vi "4wireRes.vi"(5 "Settling time":dbl=2.0, 7 "Enable Output (T: Enable)":bool, 8 "error in (no error)":errorcluster, 10 "VISA nanoVM":refnum<visa-resource-name>="nanovoltmeter", 11 "VISA current":refnum<visa-resource-name>="K2401") -> (0 "R4pt":dbl, 1 "R2pt":sgl, 2 "error out":errorcluster, 3 "VISA nanovoltmeter out":refnum<visa-resource-name>, 6 "VISA current out":refnum<visa-resource-name>)   [LabVIEW 2019]
uses:
  _Global variables 1.vi
  <instrlib>/Keithley 2182/Keithley 2182.lvlib
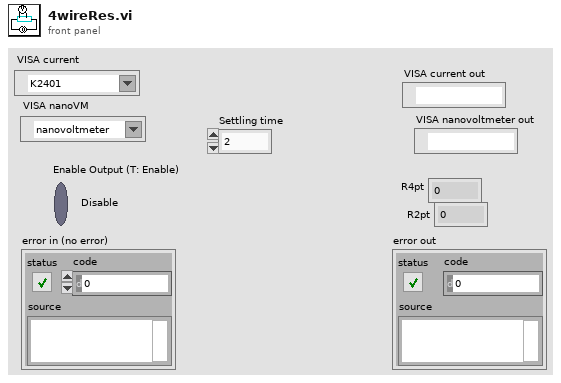
[diagram p1: front panel]
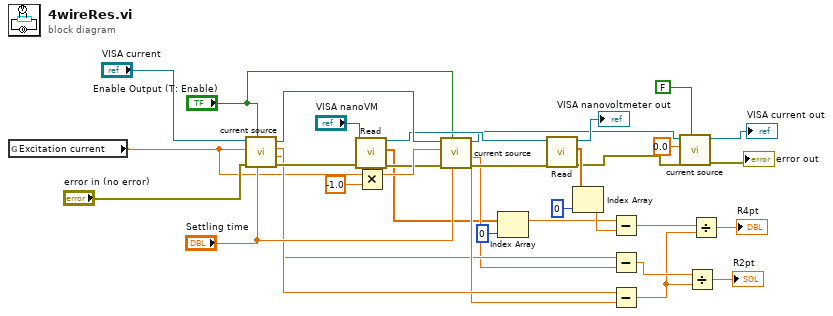
[diagram p0: block diagram]
diagram:
  n1 = global read "_Global variables 1.vi" "Excitation current"() -> (w1:dbl)
  n2 = call "current source.vi"("Settling time"="Settling time", "Enable Output (T: Enable)"="Enable Output (T: Enable)", "error in (no error)"="error in (no error)", "Output Level (0)"=w1, "VISA current"="VISA current") -> ("error out"=w33:errorcluster, "Voltage"=w22:sgl, "Current"=w24:sgl, "VISA resource name out"=w29:refnum<visa-resource-name>)  [unwired: 3 in]
  n3 = call <instrlib>:"Read.vi"("error in (no error)"=w33, "VISA resource name"="VISA nanoVM") -> ("error out"=w28:errorcluster, "Measurements"=w20:dbl[], "VISA resource name out"=w25:refnum<visa-resource-name>)  [unwired: 6 in, 1 out]
  n4 = Multiply(x=w1, y=-1.0) -> (x*y=w31:dbl)
  n5 = call "current source.vi"("Settling time"="Settling time", "Enable Output (T: Enable)"="Enable Output (T: Enable)", "error in (no error)"=w28, "Output Level (0)"=w31, "VISA current"=w29) -> ("error out"=w26:errorcluster, "Voltage"=w21:sgl, "Current"=w23:sgl, "VISA resource name out"=w7:refnum<visa-resource-name>)  [unwired: 3 in]
  n6 = Index Array(array=w20, index=0) -> (element=w15:dbl)
  n7 = call <instrlib>:"Read.vi"("error in (no error)"=w26, "VISA resource name"=w25) -> ("error out"=w5:errorcluster, "Measurements"=w19:dbl[], "VISA resource name out"=→"VISA nanovoltmeter out":refnum<visa-resource-name>)  [unwired: 6 in, 1 out]
  n8 = Index Array(array=w19, index=0) -> (element=w18:dbl)
  n9 = Subtract(x=w15, y=w18) -> (x-y=w16:dbl)
  n10 = Subtract(x=w22, y=w21) -> (x-y=w13:sgl)
  n11 = Subtract(x=w24, y=w23) -> (x-y=w12:sgl)
  n12 = call "current source.vi"("Enable Output (T: Enable)"=FALSE, "error in (no error)"=w5, "Output Level (0)"=0.0, "VISA current"=w7) -> ("error out"=→"error out":errorcluster, "VISA resource name out"=→"VISA current out":refnum<visa-resource-name>)  [unwired: 4 in, 2 out]
  n13 = Divide(x=w13, y=w12) -> (x/y=→"R2pt":sgl)
  n14 = Divide(x=w16, y=w12) -> (x/y=→"R4pt":dbl)
